vi "set engine settings.vi"(8 "error in (no error)":errorcluster, 10 "engine_settings":T1, 11 "id":i32) -> (0 "error out":errorcluster, 3 "function return":i32)   [LabVIEW 2012, in "libximc.lvlib"]
doc: "result_t XIMC_API set_engine_settings (device_t id, const engine_settings_t* engine_settings);"
uses:
  libximc.lvlib
  libximc.dll
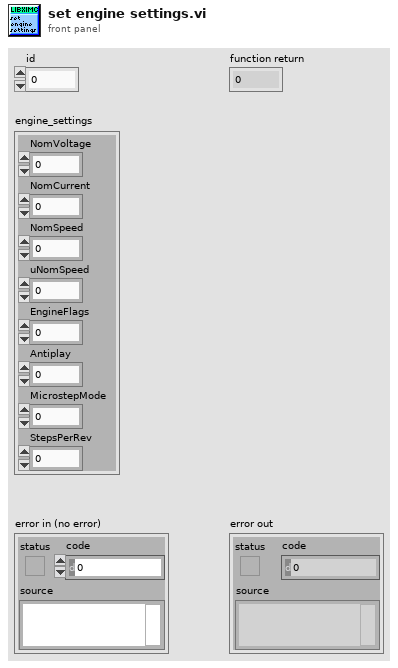
[diagram p1: front panel]
types:
  T1 = cluster{"NomVoltage":u32, "NomCurrent":u32, "NomSpeed":u32, "uNomSpeed":u32, "EngineFlags":u32, "Antiplay":i32, "MicrostepMode":u32, "StepsPerRev":u32}
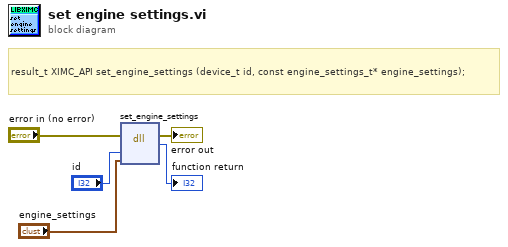
[diagram p0: block diagram]
diagram:
  # "result_t XIMC_API set_engine_settings (device_t id, const engine_settings_t* engine_settings);"
  n1 = dll-call lib="C:/Users/Stepan/Downloads/labview_2.9.11_testgen_thread/libximc.*" fn="set_engine_settings"(error in="error in (no error)", "id"="id", "engine_settings"="engine_settings") -> (error out=→"error out":errorcluster, →"function return":i32)  [unwired: 4 in, 1 out]
